vi "Send Single Trigger.vi"(8 "error in (no error)":errorcluster, 11 "VNA-Ag87xx in":refnum<class "VNA-Ag87xx.lvclass">) -> (0 "error out":errorcluster, 3 "VNA-Ag87xx out":refnum<class "VNA-Ag87xx.lvclass">)   [LabVIEW 2020, in "VNA-Ag87xx.lvclass"]
doc: "Sent a single trigger for the VNA. It uses the OPC command to wait until completion.\nIt will use (sweeptime * N average * N ports) for the VISA timeout."
uses:
  VNA-Ag87xx.lvclass
  C:/Sandbox/Git_Sandbox/WiSpry Test Framework source code (LV20)/WiSpry Test Framework/Instruments/Instrument.lvclass
  Instrument.lvclass/Instrument.ctl
  Instrument.lvclass
  <instrlib>/Agilent 87XX Series/Agilent 87XX Series.lvlib
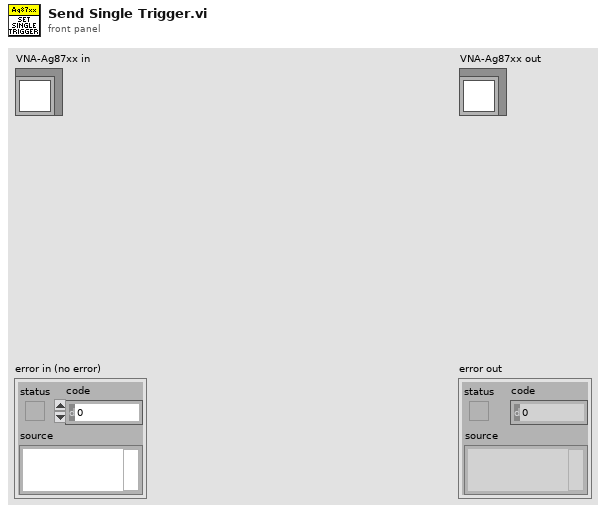
[diagram p1: front panel]
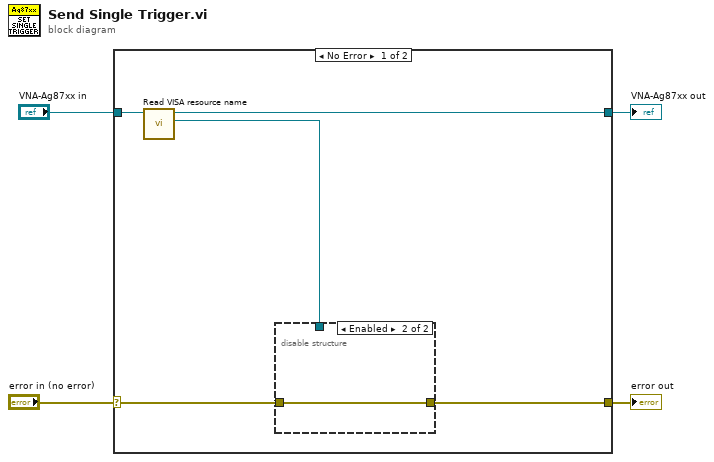
[diagram p0: block diagram]
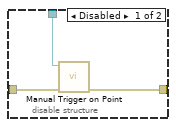
[diagram p2: hidden frame]
diagram:
  n1 = case shown="No Error" "error in (no error)" {
    selector: "error in (no error)" -> [w7 w14]
    tunnel: [w8 w15] -> w3
    tunnel: "VNA-Ag87xx in" -> [w9 w15]
    tunnel: [w6 w14] -> w1
    frame No Error {
      n2 = call "Read VISA resource name.vi"("Instrument in"=w9) -> ("VISA resource name"=w5:refnum<visa-resource-name>, "Instrument out"=w8:refnum<class "VNA-Ag87xx.lvclass">)  [unwired: 9 in]
      n3 = disable-structure shown="Enabled" {
        disable-tunnel: w7 -> [w12 w13]
        disable-tunnel: [w11 w13] -> w6
        disable-tunnel: w5 -> [w10 _]
        frame Disabled {
          n4 = call <instrlib>:"Manual Trigger on Point.vi"("error in (no error)"=w12, "VISA resource name"=w10) -> ("error out"=w11:errorcluster)  [unwired: 8 in, 1 out]
        }
        frame Enabled {
        }
      }
    }
    frame Error {
    }
  }
  "error out" <- w1
  "VNA-Ag87xx out" <- w3
